vi "track changes table.vi"(8 "error in":errorcluster, 9 "NewVal":string[][](array[string]), 10 "OldVal":string[][](array[string]), 11 "Engine Input":refnum<class "engine configuration.lvclass">) -> (0 "error out":errorcluster, 1 "change?":bool, 3 "Engine Output":refnum<class "engine configuration.lvclass">)   [LabVIEW 2013, in "PL Framework Configuration Tool.lvlib" / "EngineTags.lvclass"]
uses:
  EngineTags.lvclass
  <vilib>/NI/Module Execution Interface/Engine Configuration/engine configuration.lvclass
  <vilib>/NI/Module Execution Interface/Engine Configuration/engine configuration.lvclass/engine configuration.ctl
  <vilib>/NI/Tag Bus/tag/tag descriptor.lvclass/tag descriptor.ctl
  <vilib>/NI/Tag Bus/tag/Data Type.ctl
  <vilib>/NI/Tag Bus/tag/tag descriptor.lvclass
  <vilib>/NI/Tag Bus/tag/default value polymorphs/write default value Double.vi
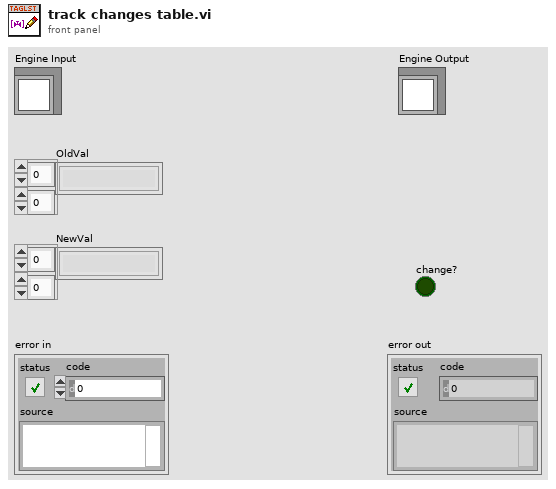
[diagram p1: front panel]
types:
  T1 = typedef "tag bus.lvlib/tag descriptor.lvclass/Data Type.ctl" = enum16{"Double", "Single", "I64", "I32", "I16", "I8", "U64", "U32", "U16", "U8", "Boolean", "String", "Array of Double", "Array of Single", "Array of I64", "Array of I32", "Array of I16", "Array of I8", "Array of U64", "Array of U32", "Array of U16", "Array of U8", "Array of Boolean", "Array of String"}
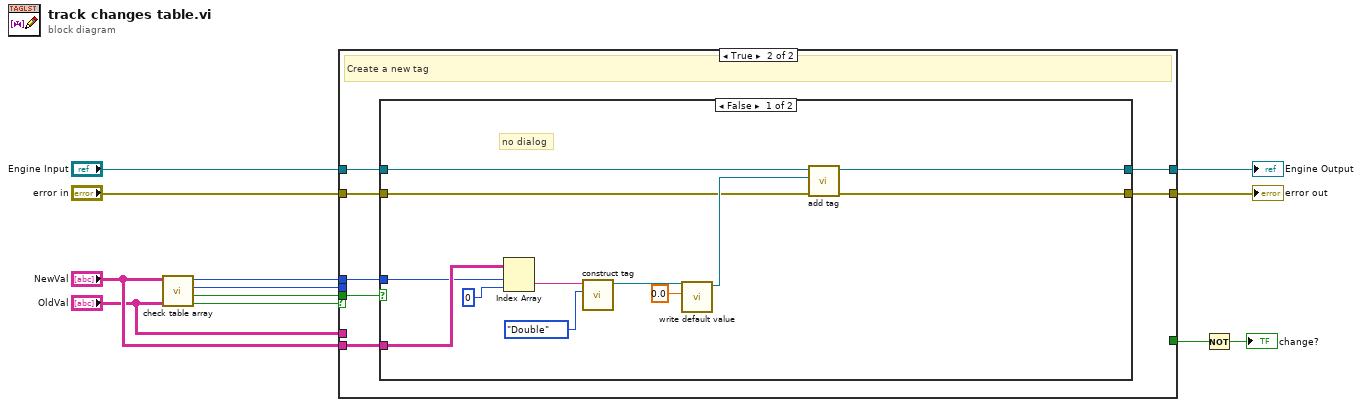
[diagram p0: block diagram]
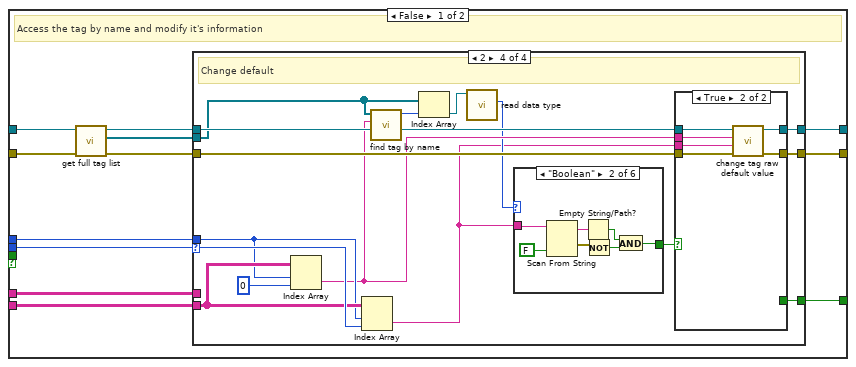
[diagram p2: hidden frame]
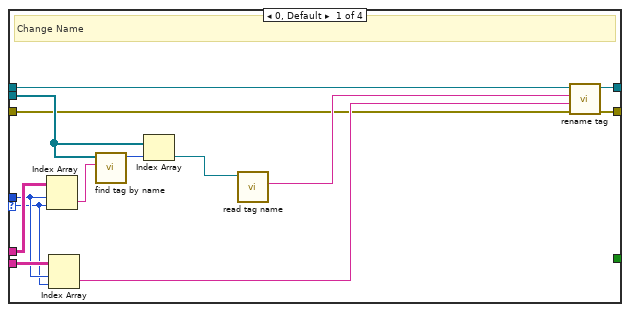
[diagram p3: hidden frame]
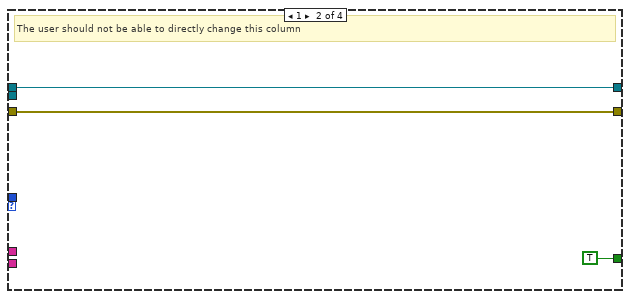
[diagram p4: hidden frame]
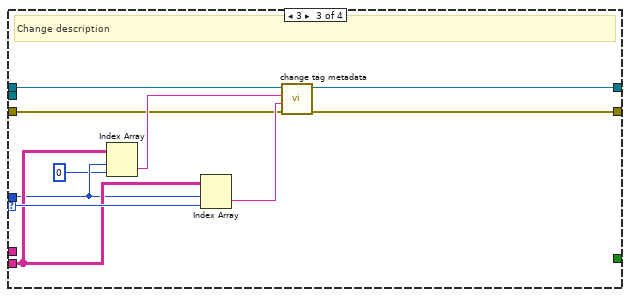
[diagram p5: hidden frame]
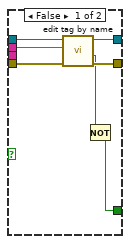
[diagram p6: hidden frame]
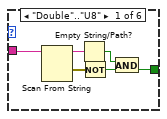
[diagram p7: hidden frame]
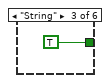
[diagram p8: hidden frame]
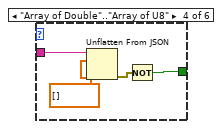
[diagram p9: hidden frame]
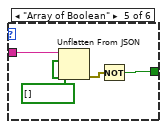
[diagram p10: hidden frame]
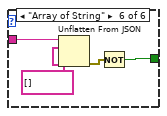
[diagram p11: hidden frame]
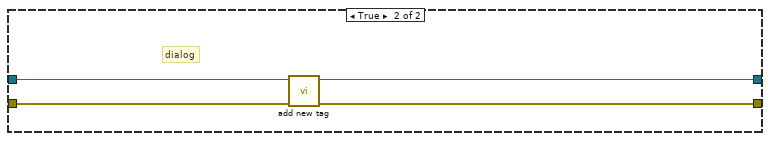
[diagram p12: hidden frame]
diagram:
  n1 = call "check table array.vi"("OldVal"="OldVal", "NewVal"="NewVal") -> ("new tag"=w6:bool, "needs dialog"=w5:bool, "Column"=w9:i32, "Row"=w10:i32)  [unwired: 6 in]
  n2 = case shown="True" w6 {
    tunnel: [w17 w109] -> w11
    tunnel: "Engine Input" -> [w21 w112]
    tunnel: "NewVal" -> [w18 w111]
    tunnel: w10 -> [w19 w110]
    tunnel: w9 -> [w23 _]
    tunnel: "OldVal" -> [w20 _]
    tunnel: w5 -> [_ w108]
    tunnel: "error in" -> [w15 w107]
    tunnel: [w14 w106] -> w3
    tunnel: [w13 _] -> w2
    frame False {
      # "Access the tag by name and modify it's information"
      n3 = call <vilib>:"get full tag list.vi"("engine configuration in"=w21) -> ("tag list"=w22:refnum<class "tag descriptor.lvclass">[], "engine configuration out"=w16:refnum<class "engine configuration.lvclass">)  [unwired: 9 in]
      n4 = case shown="2" w23 {
        selector: w23 -> [w33 _ w48 w66]
        tunnel: w22 -> [w29 _ _ w57]
        tunnel: w20 -> [w37 _ _ _]
        tunnel: w19 -> [w34 _ w46 w64]
        tunnel: w18 -> [w35 _ w47 w65]
        tunnel: [w31 w40 w49 w61] -> w17
        tunnel: w16 -> [w30 w40 w50 w62]
        tunnel: w15 -> [w25 w39 w42 w59]
        tunnel: [w24 w39 w41 w60] -> w14
        tunnel: [_ TRUE _ w51] -> w13
        frame 0, Default {
          # "Change Name"
          n5 = Index Array(array=w37, index (row)=w34, index (col)=w33) -> (element=w36:string)
          n6 = Index Array(array=w35, index (row)=w34, index (col)=w33) -> (element=w32:string)
          n7 = call <vilib>:"find tag by name.vi"("name"=w36, "tags in"=w29) -> ("index"=w27:i32)  [unwired: 9 in]
          n8 = Index Array(array=w29, index=w27) -> (element=w28:refnum<class "tag descriptor.lvclass">)
          n9 = call <vilib>:"read tag name.vi"("system tag in"=w28) -> ("name"=w26:string)  [unwired: 8 in, 2 out]
          n10 = call <vilib>:"rename tag.vi"("error in"=w25, "new name"=w32, "old name"=w26, "engine configuration in"=w30) -> ("error out"=w24:errorcluster, "engine configuration out"=w31:refnum<class "engine configuration.lvclass">)  [unwired: 6 in]
        }
        frame 1 {
          # "The user should not be able to directly change this column"
        }
        frame 3 {
          # "Change description"
          n11 = Index Array(array=w47, index (row)=w46, index (col)=0 ("disabled index (col)")) -> (element=w45:string)
          n12 = Index Array(array=w47, index (row)=w46, index (col)=w48) -> (element=w44:string)
          n13 = call <vilib>:"change tag metadata.vi"("error in"=w42, "metadata"=w44, "tag name"=w45, "engine configuration in"=w50) -> ("error out"=w41:errorcluster, "engine configuration out"=w49:refnum<class "engine configuration.lvclass">)  [unwired: 6 in]
        }
        frame 2 {
          # "Change default"
          n14 = Index Array(array=w65, index (row)=w64, index (col)=0 ("disabled index (col)")) -> (element=w56:string)
          n15 = Index Array(array=w65, index (row)=w64, index (col)=w66) -> (element=w53:string)
          n16 = call <vilib>:"find tag by name.vi"("name"=w56, "tags in"=w57) -> ("index"=w58:i32)  [unwired: 9 in]
          n17 = Index Array(array=w57, index=w58) -> (element=w55:refnum<class "tag descriptor.lvclass">)
          n18 = call <vilib>:"read data type.vi"("system tag in"=w55) -> ("data type"=w54:T1)  [unwired: 8 in, 2 out]
          n19 = case shown="\"Boolean\"" w54 {
            tunnel: w53 -> [w85 w92 _ w97 w101 w105]
            tunnel: [w81 w86 TRUE w94 w98 w102] -> w52
            frame "Double".."U8" {
              n20 = Scan From String(input string=w85) -> (remaining string=w82:string, error out=w84:errorcluster)  [unwired: 5 in, 1 out]
              n21 = Empty String/Path?(string/path=w82) -> (empty?=w80:bool)
              n22 = Not(x=w84) -> (.not. x?=w83:bool)
              n23 = And(x=w80, y=w83) -> (x .and. y?=w81:bool)
            }
            frame "Boolean" {
              n24 = Scan From String(input string=w92, default 1=FALSE) -> (remaining string=w87:string, error out=w88:errorcluster)  [unwired: 4 in, 1 out]
              n25 = Empty String/Path?(string/path=w87) -> (empty?=w89:bool)
              n26 = Not(x=w88) -> (.not. x?=w90:bool)
              n27 = And(x=w89, y=w90) -> (x .and. y?=w86:bool)
            }
            frame "String" {
            }
            frame "Array of Double".."Array of U8" {
              n28 = Unflatten From JSON(JSON string=w97, type and defaults=dbl[] []) -> (error out=w95:errorcluster)  [unwired: 5 in, 1 out]
              n29 = Not(x=w95) -> (.not. x?=w94:bool)
            }
            frame "Array of Boolean" {
              n30 = Unflatten From JSON(JSON string=w101, type and defaults=bool[] []) -> (error out=w99:errorcluster)  [unwired: 5 in, 1 out]
              n31 = Not(x=w99) -> (.not. x?=w98:bool)
            }
            frame "Array of String" {
              n32 = Unflatten From JSON(JSON string=w105, type and defaults=string[] []) -> (error out=w103:errorcluster)  [unwired: 5 in, 1 out]
              n33 = Not(x=w103) -> (.not. x?=w102:bool)
            }
          }
          n34 = case shown="True" w52 {
            tunnel: w62 -> [w73 w79]
            tunnel: [w70 w78] -> w61
            tunnel: [w69 w77] -> w60
            tunnel: w59 -> [w72 w76]
            tunnel: w56 -> [w71 w75]
            tunnel: w53 -> [_ w74]
            tunnel: [w67 _] -> w51
            frame False {
              n35 = call "edit tag by name.vi"("error in"=w72, "name"=w71, "engine configuration in"=w73) -> ("error out"=w69:errorcluster, "change?"=w68:bool, "engine configuration out"=w70:refnum<class "engine configuration.lvclass">)  [unwired: 6 in]
              n36 = Not(x=w68) -> (.not. x?=w67:bool)
            }
            frame True {
              n37 = call <vilib>:"change tag raw default value.vi"("error in"=w76, "raw default"=w74, "tag name"=w75, "engine configuration in"=w79) -> ("error out"=w77:errorcluster, "engine configuration out"=w78:refnum<class "engine configuration.lvclass">)  [unwired: 6 in]
            }
          }
        }
      }
    }
    frame True {
      # "Create a new tag"
      n38 = case shown="False" w108 {
        tunnel: w112 -> [w124 w128]
        tunnel: w111 -> [w123 _]
        tunnel: w110 -> [w122 _]
        tunnel: [w118 w126] -> w109
        tunnel: w107 -> [w114 w127]
        tunnel: [w113 w125] -> w106
        frame False {
          # "no dialog"
          n39 = Index Array(array=w123, index (row)=w122, index (col)=0 ("disabled index (col)")) -> (element=w120:string)
          n40 = call <vilib>:"construct tag.vi"("data type"=Data_Type."Double", "name"=w120) -> ("system tag out"=w117:refnum<class "tag descriptor.lvclass">)  [unwired: 8 in, 1 out]
          n41 = call-poly <vilib>:"write default value.vi"("default value"=0.0, "system tag in"=w117) -> ("system tag out"=w116:refnum<class "tag descriptor.lvclass">)  [unwired: 8 in, 1 out]
          n42 = call <vilib>:"add tag.vi"("error in"=w114, "tag descriptor"=w116, "engine configuration in"=w124) -> ("error out"=w113:errorcluster, "engine configuration out"=w118:refnum<class "engine configuration.lvclass">)  [unwired: 7 in]
        }
        frame True {
          # "dialog"
          n43 = call "add new tag.vi"("error in"=w127, "engine configuration in"=w128) -> ("error out"=w125:errorcluster, "engine configuration out"=w126:refnum<class "engine configuration.lvclass">)  [unwired: 8 in]
        }
      }
    }
  }
  "error out" <- w3
  "Engine Output" <- w11
  n44 = Not(x=w2) -> (.not. x?=→"change?":bool)
